vi "getDataTypeTel.vi"(8 "error in (no error)":errorcluster, 10 "name":string, 11 "LibReader in":refnum<class "LibReader.lvclass">) -> (0 "error out":errorcluster, 2 "pathDataType":path, 3 "LibReader out":refnum<class "LibReader.lvclass">)   [LabVIEW 2018, in "LibReader.lvclass"]
doc: "Get the data type of telemetry."
uses:
  LibReader.lvclass
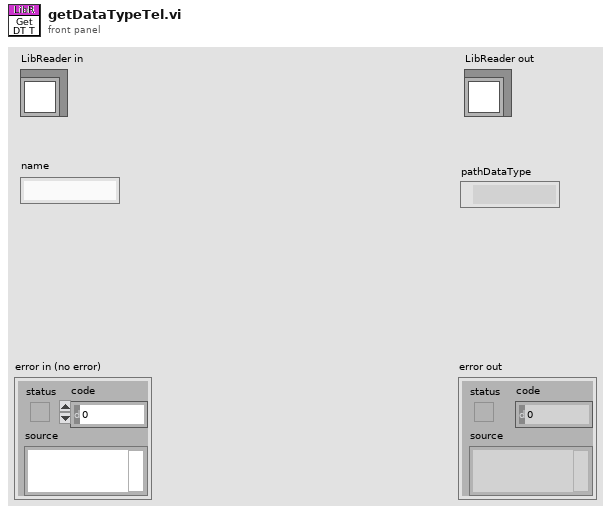
[diagram p1: front panel]
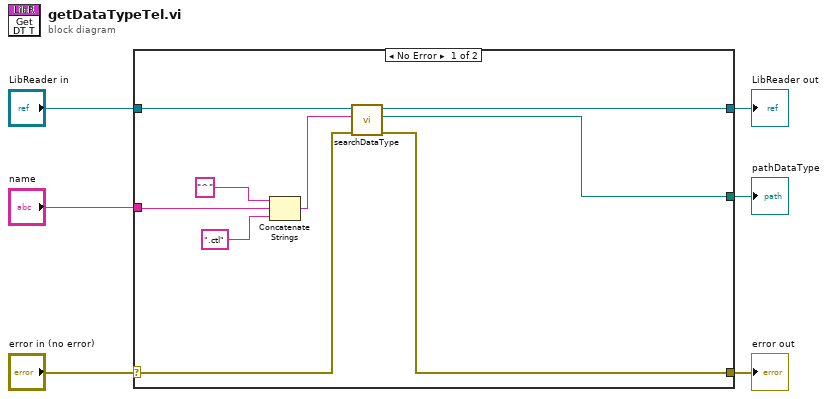
[diagram p0: block diagram]
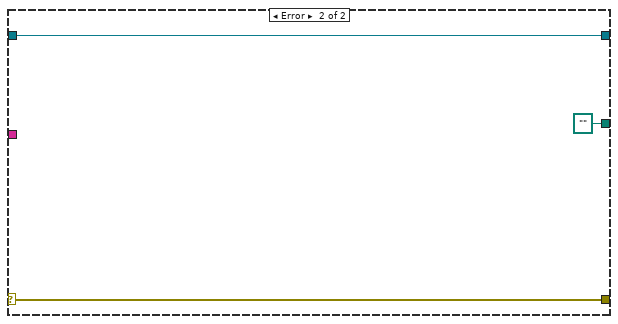
[diagram p2: hidden frame]
diagram:
  n1 = case shown="No Error" "error in (no error)" {
    selector: "error in (no error)" -> [w12 w18]
    tunnel: [w11 w18] -> w5
    tunnel: [w14 w17] -> w3
    tunnel: "LibReader in" -> [w15 w17]
    tunnel: [w13 path "" ("pathDataType")] -> w2
    tunnel: "name" -> [w9 _]
    frame No Error {
      n2 = Concatenate Strings("^", w9, ".ctl" ("regExpr")) -> (w8:string)
      n3 = call "searchDataType.vi"("error in (no error)"=w12, "regExpr"=w8, "LibReader in"=w15) -> ("error out"=w11:errorcluster, "pathDataType"=w13:path, "LibReader out"=w14:refnum<class "LibReader.lvclass">)  [unwired: 6 in]
    }
    frame Error {
    }
  }
  "error out" <- w5
  "LibReader out" <- w3
  "pathDataType" <- w2
